vi "Add Cell Format.vi"(8 "error in":errorcluster, 10 "Font Id":i32=-1, 11 "SpreadsheetDoc in":refnum<k24>) -> (0 "error out":errorcluster, 2 "Style Index":u32, 3 "SpreadsheetDoc out":refnum<k24>)   [LabVIEW 2021, in "Open Xml.lvlib"]
uses:
  Open Xml.lvlib
  D:/git/Open-Xml-LabVIEW/dll/DocumentFormat.OpenXml.dll
  dll/DocumentFormat.OpenXml.dll
  D:/git/Open-Xml-LabVIEW/dll/DocumentFormat.OpenXml.Framework.dll
  dll/DocumentFormat.OpenXml.Framework.dll
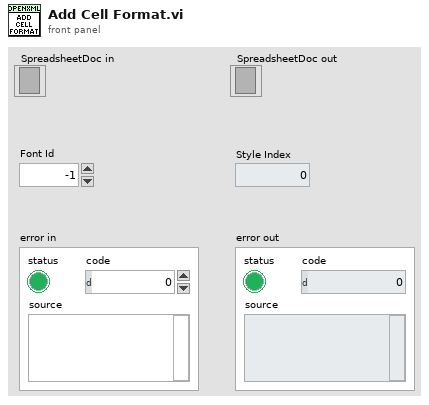
[diagram p1: front panel]
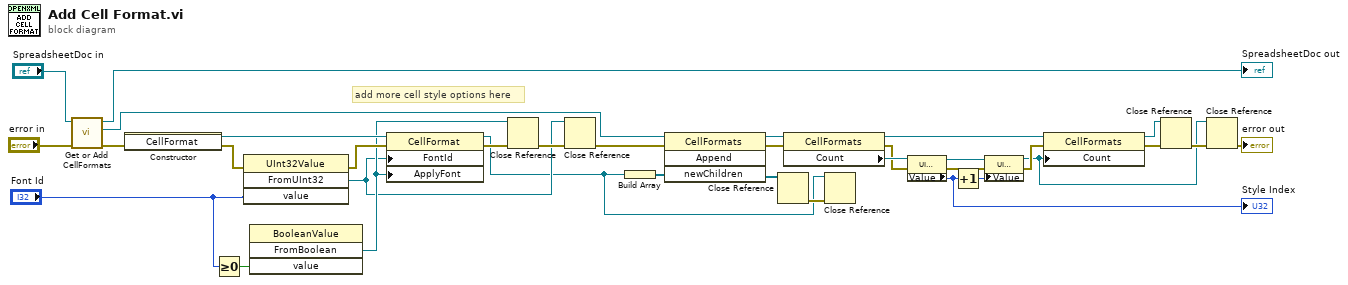
[diagram p0: block diagram]
diagram:
  # "add more cell style options here"
  n1 = call "Get or Add CellFormats.vi"("error in"="error in", "SpreadsheetDoc in"="SpreadsheetDoc in") -> ("error out"=w32:errorcluster, "CellFormats"=w24:refnum<k24>, "SpreadsheetDoc out"=→"SpreadsheetDoc out":refnum<k24>)  [unwired: 7 in]
  n2 = constructor class="CellFormat"(error in=w32) -> (reference out=w34:refnum<k24>, error out=w28:errorcluster)  [unwired: 2 in, 1 out]
  n3 = Greater Or Equal To 0?(x="Font Id") -> (x >= 0?=w26:bool)
  n4 = invoke class="UInt32Value" method="FromUInt32"(error in=w28, "value"="Font Id") -> (error out=w27:errorcluster, "FromUInt32"=w8:refnum<k24>)  [unwired: 2 in, 2 out]
  n5 = invoke class="BooleanValue" method="FromBoolean"("value"=w26) -> ("FromBoolean"=w9:refnum<k24>)  [unwired: 3 in, 3 out]
  n6 = property class="CellFormat"(reference=w34, error in=w27, "FontId"=w8, "ApplyFont"=w9) -> (reference out=w3:refnum<k24>, error out=w29:errorcluster)
  n7 = Close Reference(reference=w9, error in (no error)=w29) -> (error out=w11:errorcluster)
  n8 = Close Reference(reference=w8, error in (no error)=w11) -> (error out=w10:errorcluster)
  n9 = Build Array(w3) -> (w7:refnum<k24>[])
  n10 = invoke class="CellFormats" method="Append"(reference=w24, error in=w10, "newChildren"=w7) -> (reference out=w23:refnum<k24>, error out=w5:errorcluster, "newChildren"=w6:refnum<k24>[])  [unwired: 1 in, 1 out]
  n11 = Close Reference(reference=w6) -> (error out=w4:errorcluster)  [unwired: 1 in]
  n12 = property class="CellFormats"(reference=w23, error in=w5) -> (reference out=w21:refnum<k24>, error out=w16:errorcluster, "Count"=w20:refnum<k24>)
  n13 = Close Reference(reference=w3, error in (no error)=w4) -> ()  [unwired: 1 out]
  n14 = property class="UInt32Value"(reference=w20, error in=w16) -> (reference out=w19:refnum<k24>, error out=w17:errorcluster, "Value"=w14:u32)
  "Style Index" <- w14
  n15 = Increment(x=w14) -> (x+1=w18:u32)
  n16 = property class="UInt32Value"(reference=w19, error in=w17, "Value"=w18) -> (reference out=w1:refnum<k24>, error out=w15:errorcluster)
  n17 = property class="CellFormats"(reference=w21, error in=w15, "Count"=w1) -> (reference out=w12:refnum<k24>, error out=w22:errorcluster)
  n18 = Close Reference(reference=w12, error in (no error)=w22) -> (error out=w13:errorcluster)
  n19 = Close Reference(reference=w1, error in (no error)=w13) -> (error out=→"error out":errorcluster)
